vi "Function Generator.vi"(8 "error in (no error)":errorcluster, 11 "Function Generator in":refnum<class "Function Generator.lvclass">) -> (0 "error out":errorcluster, 3 "Function Generator out":refnum<class "Function Generator.lvclass">)   [LabVIEW 2017, in "Function Generator.lvclass"]
uses:
  Function Generator.lvclass
  Global/GPIB Numbers.vi
panel:
  out "Status":string
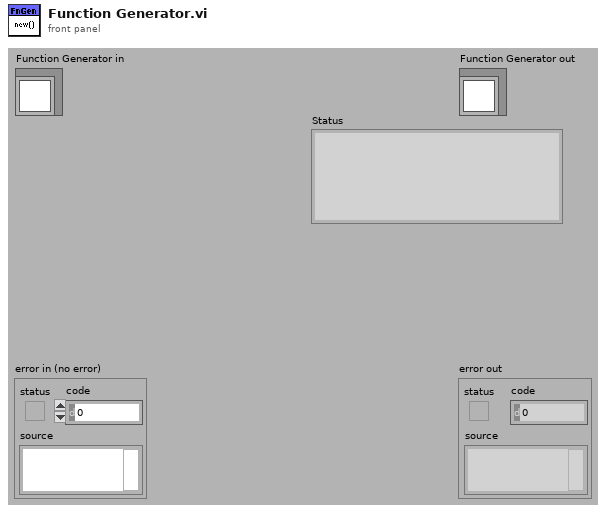
[diagram p1: front panel]
types:
  T1 = typedef "GPIB Type Def.ctl" = cluster{"Name":string, "bus":dbl, "GPIB":dbl, "GPIB as string":string, "byte":i32, "VISA Resource Name":refnum<visa-resource-name>}
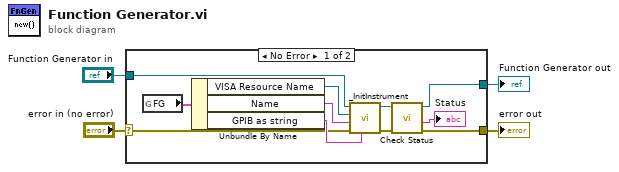
[diagram p0: block diagram]
diagram:
  n1 = case shown="No Error" "error in (no error)" {
    selector: "error in (no error)" -> [w11 w17]
    tunnel: [w6 w17] -> w3
    tunnel: [w8 w16] -> w1
    tunnel: "Function Generator in" -> [w10 w16]
    frame No Error {
      n2 = global read "GPIB Numbers.vi" "FG"() -> (w15:T1)
      n3 = Unbundle By Name(w15) -> ("VISA Resource Name"=w14:refnum<visa-resource-name>, "Name"=w13:string, "GPIB as string"=w12:string)
      n4 = call-dynamic "_InitInstrument.vi"("GPIB as string"=w12, "error in (no error)"=w11, "Name"=w13, "VISA Resource Name"=w14, "Instrument in"=w10) -> ("error out"=w7:errorcluster, "Instrument out"=w9:refnum<class "Function Generator.lvclass">)  [unwired: 1 in, 4 out]
      n5 = call-dynamic "Check Status.vi"("error in (no error)"=w7, "Function Generator in"=w9) -> ("error out"=w6:errorcluster, "Status"=→"Status":string, "Function Generator out"=w8:refnum<class "Function Generator.lvclass">)  [unwired: 7 out]
    }
    frame Error {
    }
  }
  "error out" <- w3
  "Function Generator out" <- w1
